vi "Data_Acquisition.vi"(11 "Error_In":errorcluster) -> (15 "Error_Out":errorcluster)   [LabVIEW 2021]
doc: "This VI Generate or simulate the data and transfer to MainVI."
uses:
  <vilib>/numeric/Random Number (Range) DBL.vi
  Controls/Generated_data.ctl
  Controls/Queue_Operation_Select.ctl
  Controls/State_and_Data.ctl
  Controls/Timer_Select.ctl
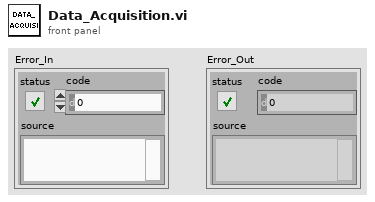
[diagram p1: front panel]
types:
  T1 = typedef "Timer_Select.ctl" = enum16{"Start_Timer", "Time_Out?", "Stop_Timer"}
  T2 = typedef "State_and_Data.ctl" = cluster{"State":string, "Data":variant}
  T3 = typedef "Queue_Operation_Select.ctl" = enum16{"Obtain_Queue", "Enqueue", "Enqueue_First", "Enqueue_N", "Lossy_Enqueue", "Preview", "Queue_Status", "Dequeue", "Flush", "Release_Queue"}
  T4 = typedef "Generated_data.ctl" = cluster{"Current_Data":dbl, "Temp_Data":dbl}
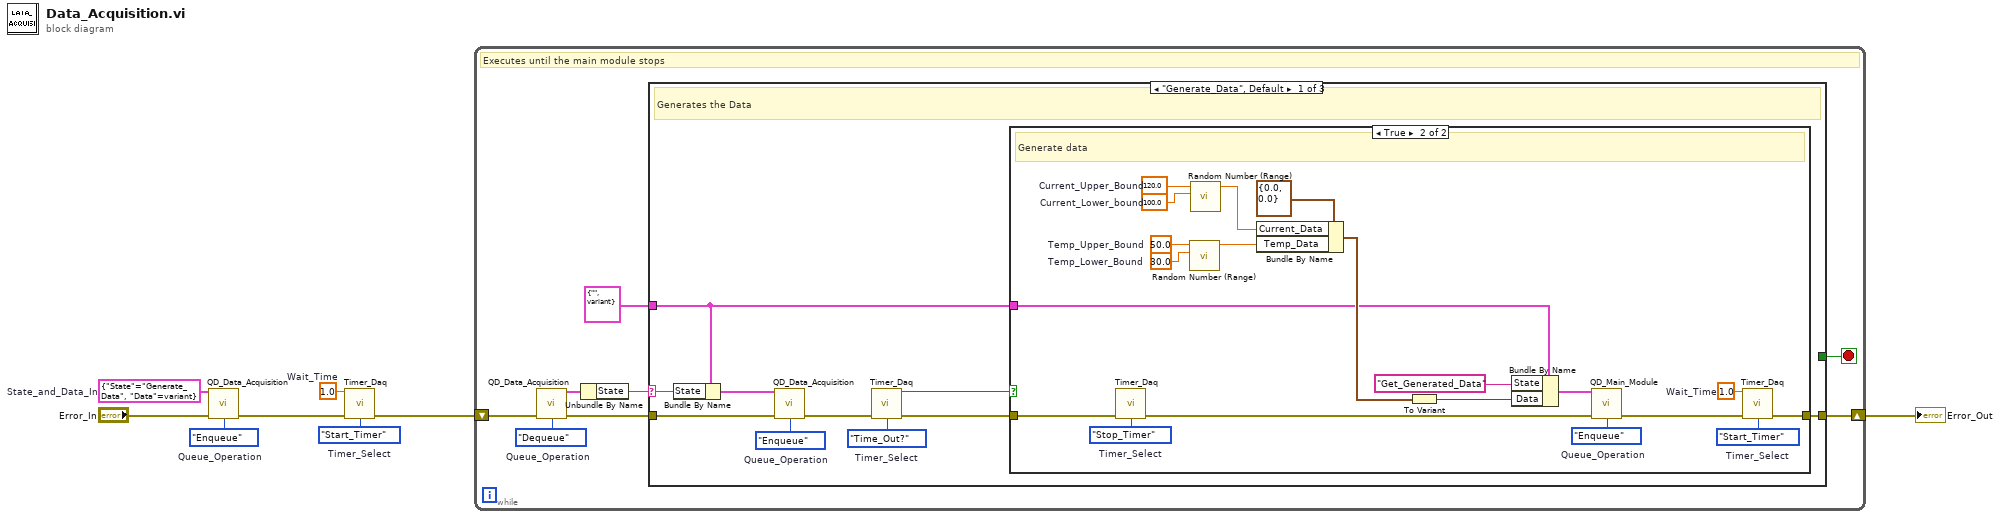
[diagram p0: block diagram]
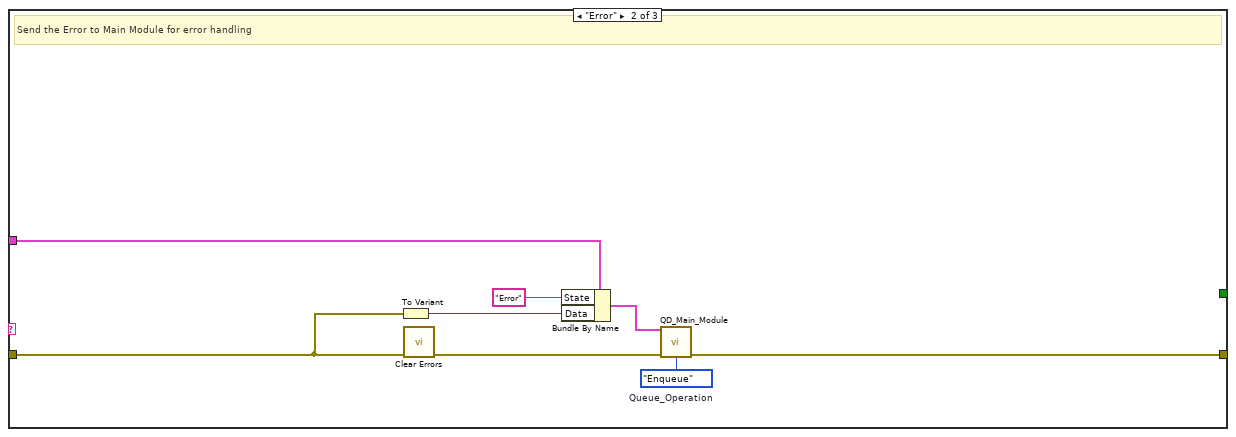
[diagram p3: hidden frame]
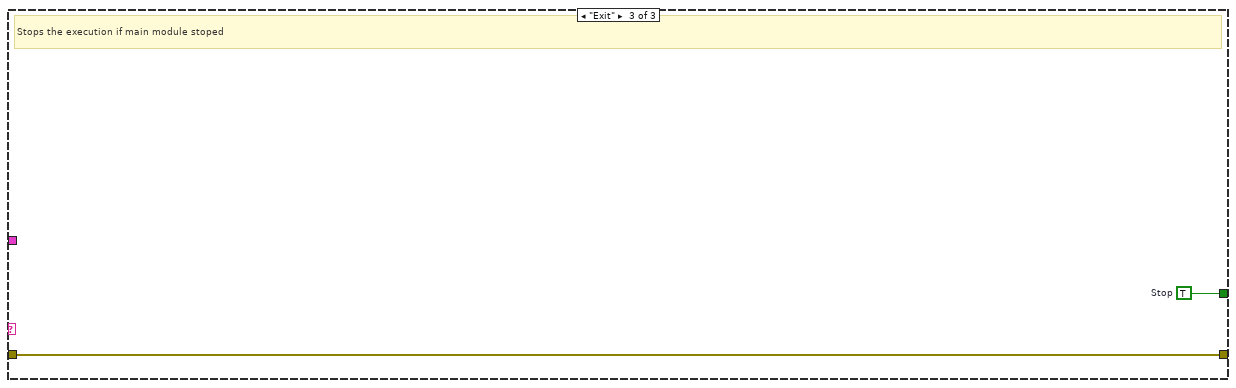
[diagram p4: hidden frame]
diagram:
  w2 = 1.0  # Wait_Time
  w3 = Timer_Select."Start_Timer"  # Timer_Select
  w5 = T2 {"State"="Generate_Data", "Data"=variant}  # State_and_Data_In
  w6 = Queue_Operation_Select."Enqueue"  # Queue_Operation
  n1 = call "QD_Data_Acquisition.vi"("State_and_Data_In"=w5, "Error_In"="Error_In", "Queue_Operation"=w6) -> ("Error_Out"=w7:errorcluster)  [unwired: 10 in, 2 out]
  n2 = call "Timer_Daq.vi"("Wait_Time"=w2, "Error_In"=w7, "Timer_Select"=w3) -> ("Error_Out"=w4:errorcluster)  [unwired: 11 in, 1 out]
  n3 = while {
    shift-right: [w16] -> w1
    shift-left: w4 -> [w15]
    stop <- w12 stop-if-true
    w10 = Queue_Operation_Select."Dequeue"  # Queue_Operation
    # "Executes until the main module stops"
    n4 = call "QD_Data_Acquisition.vi"("Error_In"=w15, "Queue_Operation"=w10) -> ("State_and_Data_Out"=w9:T2, "Error_Out"=w14:errorcluster)  [unwired: 11 in, 1 out]
    n5 = Unbundle By Name(w9) -> ("State"=w13:string)
    n6 = case shown="\"Generate_Data\", Default" w13 {
      selector: w13 -> [w18 _ _]
      tunnel: w14 -> [w20 w48 w57]
      tunnel: [w26 w55 w57] -> w16
      tunnel: [_ _ w56] -> w12
      tunnel: T2 {"State"="", "Data"=variant} ("Data_In") -> [w17 w53 _]
      frame "Generate_Data", Default {
        w21 = Queue_Operation_Select."Enqueue"  # Queue_Operation
        w23 = Timer_Select."Time_Out?"  # Timer_Select
        # "Generates the Data"
        n7 = Bundle By Name(cluster=w17, "State"=w18) -> (w22:T2)
        n8 = call "QD_Data_Acquisition.vi"("State_and_Data_In"=w22, "Error_In"=w20, "Queue_Operation"=w21) -> ("Error_Out"=w19:errorcluster)  [unwired: 10 in, 2 out]
        n9 = call "Timer_Daq.vi"("Error_In"=w19, "Timer_Select"=w23) -> ("Time_Out?"=w24:bool, "Error_Out"=w25:errorcluster)  [unwired: 12 in]
        n10 = case shown="True" w24 {
          tunnel: w25 -> [w27 w40]
          tunnel: [w27 w31] -> w26
          tunnel: w17 -> [_ w33]
          frame False {
          }
          frame True {
            w29 = 1.0  # Wait_Time
            w30 = Timer_Select."Start_Timer"  # Timer_Select
            w32 = Timer_Select."Stop_Timer"  # Timer_Select
            w35 = Queue_Operation_Select."Enqueue"  # Queue_Operation
            w44 = 30.0  # Temp_Lower_Bound
            w45 = 50.0  # Temp_Upper_Bound
            w46 = 100.0  # Current_Lower_bound
            w47 = 120.0  # Current_Upper_Bound
            # "Generate data"
            n11 = call "Timer_Daq.vi"("Error_In"=w40, "Timer_Select"=w32) -> ("Error_Out"=w28:errorcluster)  [unwired: 12 in, 1 out]
            n12 = call-poly <vilib>:"Random Number (Range).vi"("lower bound (0)"=w44, "upper bound (100)"=w45) -> ("number"=w42:dbl)  [unwired: 9 in]
            n13 = call-poly <vilib>:"Random Number (Range).vi"("lower bound (0)"=w46, "upper bound (100)"=w47) -> ("number"=w43:dbl)  [unwired: 9 in]
            n14 = Bundle By Name(cluster=T4 {"Current_Data"=0.0, "Temp_Data"=0.0} ("Generated_Data"), "Current_Data"=w43, "Temp_Data"=w42) -> (w38:T4)
            n15 = To Variant(anything=w38) -> (Variant=w37:variant)
            n16 = Bundle By Name(cluster=w33, "State"="Get_Generated_Data", "Data"=w37) -> (w39:T2)
            n17 = call "QD_Main_Module.vi"("Data_In"=w39, "Error_In"=w28, "Queue_Operation"=w35) -> ("Error_Out"=w34:errorcluster)  [unwired: 10 in, 2 out]
            n18 = call "Timer_Daq.vi"("Wait_Time"=w29, "Error_In"=w34, "Timer_Select"=w30) -> ("Error_Out"=w31:errorcluster)  [unwired: 11 in, 1 out]
          }
        }
      }
      frame "Error" {
        w54 = Queue_Operation_Select."Enqueue"  # Queue_Operation
        # "Send the Error to Main Module for error handling"
        n19 = To Variant(anything=w48) -> (Variant=w50:variant)
        n20 = call <vilib>:"Clear Errors.vi"("error in (no error)"=w48) -> ("error out"=w49:errorcluster)  [unwired: 5 in, 1 out]
        n21 = Bundle By Name(cluster=w53, "State"="Error", "Data"=w50) -> (w52:T2)
        n22 = call "QD_Main_Module.vi"("Data_In"=w52, "Error_In"=w49, "Queue_Operation"=w54) -> ("Error_Out"=w55:errorcluster)  [unwired: 10 in, 2 out]
      }
      frame "Exit" {
        w56 = TRUE  # Stop
        # "Stops the execution if main module stoped"
      }
    }
  }
  "Error_Out" <- w1
